vi "Revision Query.vi"(8 "error in (no error)":errorcluster, 11 "VISA resource name":refnum<visa-resource-name>) -> (0 "error out":errorcluster, 1 "Instrument Firmware Revision":string, 2 "Instrument Driver Revision":string, 3 "VISA resource name out":refnum<visa-resource-name>)   [LabVIEW 2018, in "XP Power PLS600.lvlib"]
doc: "Queries the current instrument firmware revision and instrument driver revision.\n\nRefer to the Readme file for detailed driver information including modification history."
uses:
  XP Power PLS600.lvlib
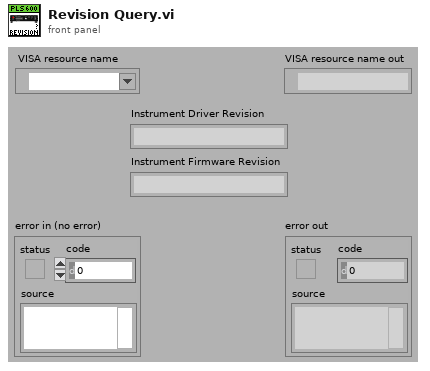
[diagram p1: front panel]
types:
  T1 = cluster{"Major":u16, "Minor":u16, "Fix":u16, "Build":u16}
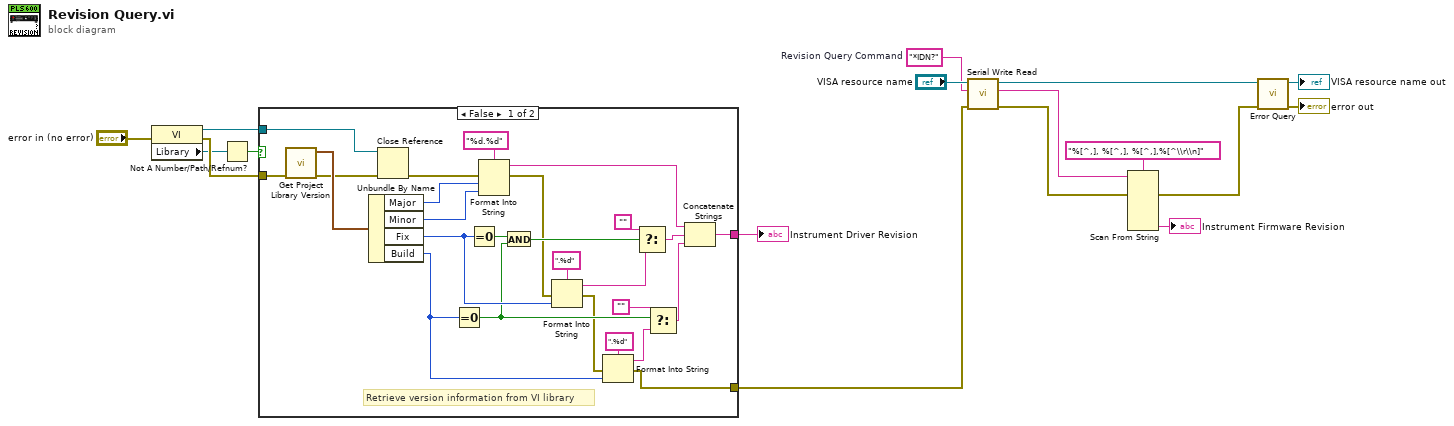
[diagram p0: block diagram]
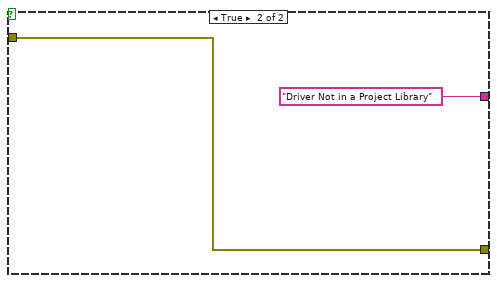
[diagram p2: hidden frame]
diagram:
  w1 = "*IDN?"  # Revision Query Command
  n1 = property class="VI"(error in="error in (no error)") -> (reference out=w11:refnum<vi>, error out=w10:errorcluster, "Library"=w9:refnum<vi>)  [unwired: 1 in]
  n2 = Not A Number/Path/Refnum?(number/path/refnum=w9) -> (NaN/Path/Refnum?=w8:bool)
  n3 = case shown="False" w8 {
    tunnel: w11 -> [w43 _]
    tunnel: w10 -> [w24 w44]
    tunnel: [w25 "Driver Not in a Project Library"] -> w13
    tunnel: [w18 w44] -> w6
    frame False {
      # "Retrieve version information from VI library"
      n4 = call <vilib>:"Get Project Library Version.vi"("error in (no error)"=w24) -> ("error out"=w22:errorcluster, "Project Library Version"=w23:T1)  [unwired: 9 in]
      n5 = Unbundle By Name(w23) -> ("Major"=w32:u16, "Minor"=w31:u16, "Fix"=w29:u16, "Build"=w30:u16)
      n6 = Close Reference(reference=w43, error in (no error)=w22) -> (error out=w21:errorcluster)
      n7 = Equal To 0?(x=w30) -> (x = 0?=w27:bool)
      n8 = Equal To 0?(x=w29) -> (x = 0?=w28:bool)
      n9 = Format Into String(format string="%d.%d", error in=w21, w32, w31) -> (resulting string=w38:string, error out=w20:errorcluster)  [unwired: 1 in]
      n10 = And(x=w28, y=w27) -> (x .and. y?=w26:bool)
      n11 = Format Into String(format string=".%d", error in=w20, w29) -> (resulting string=w40:string, error out=w19:errorcluster)  [unwired: 1 in]
      n12 = Format Into String(format string=".%d", error in=w19, w30) -> (resulting string=w36:string, error out=w18:errorcluster)  [unwired: 1 in]
      n13 = Select(t="", s=w26, f=w40) -> (s? t:f=w37:string)
      n14 = Select(t="", s=w27, f=w36) -> (s? t:f=w33:string)
      n15 = Concatenate Strings(w38, w37, w33) -> (w25:string)
    }
    frame True {
    }
  }
  "Instrument Driver Revision" <- w13
  n16 = call "Serial Write Read.vi"("error in (no error)"=w6, "Write Buffer"=w1, "VISA resource name"="VISA resource name") -> ("error out"=w5:errorcluster, "Read Buffer"=w4:string, "VISA resource name out"=w3:refnum<visa-resource-name>)  [unwired: 6 in]
  n17 = Scan From String(format string="%[^,], %[^,], %[^,],%[^\\r\\n]", input string=w4, error in=w5) -> (error out=w7:errorcluster, output 4=→"Instrument Firmware Revision":string)  [unwired: 8 in, 2 out]
  n18 = call "Error Query.vi"("error in (no error)"=w7, "VISA resource name"=w3) -> ("error out"=→"error out":errorcluster, "VISA resource name out"=→"VISA resource name out":refnum<visa-resource-name>)  [unwired: 6 in, 2 out]
